vi "motor set direction.vi"(8 "error in (no error)":errorcluster, 10 "direction":enum16{"counter-clockwise", "clockwise"}(ring), 11 "Handle In":i32) -> (0 "error out":errorcluster, 3 "Handle Out":i32)   [LabVIEW 2013]
uses:
  motor constants.ctl
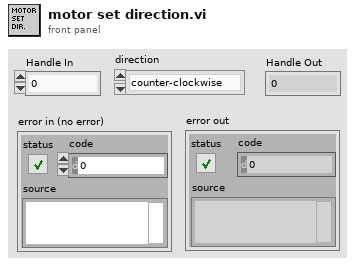
[diagram p1: front panel]
types:
  T1 = typedef "motor constants.ctl" = u16
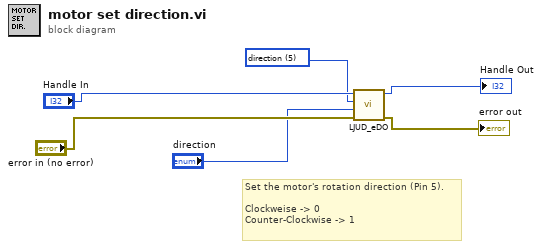
[diagram p0: block diagram]
diagram:
  w2 = T1 5 items=["enable"=4, "direction"=5, "step"=6, "end switch"=7] ("motor pin settings")
  # "Set the motor's rotation direction (Pin 5).\n\nClockweise -> 0\nCounter-Clockwise -> 1"
  n1 = call <vilib>:"LJUD_eDO.vi"("error in"="error in (no error)", "State"="direction", "Channel"=w2, "Handle In"="Handle In") -> ("error out"=→"error out":errorcluster, "Handle Out"=→"Handle Out":i32)  [unwired: 6 in]
